vi "TextControlledInstrumCommandsToArraySingle.vi"(10 "SetGetCommands":string, 11 "Control":refnum<vi>) -> (2 "Control to Index":T1(c390), 3 "Command Array":string[][](array[string]))   [LabVIEW 2019]
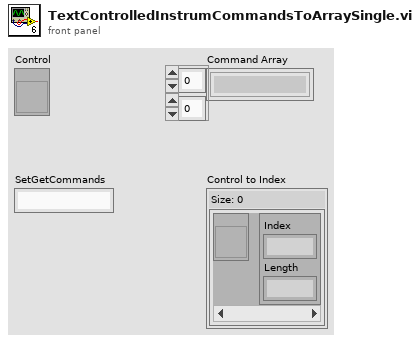
[diagram p1: front panel]
types:
  T1 = map{refnum<vi>, cluster{"Index":i32, "Length":i32}}
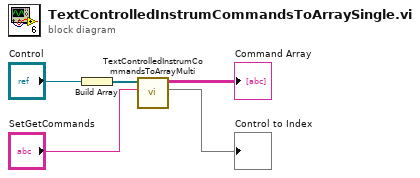
[diagram p0: block diagram]
diagram:
  n1 = Build Array("Control") -> (w4:refnum<vi>[])
  n2 = call "TextControlledInstrumCommandsToArrayMulti.vi"("SetGetCommands"="SetGetCommands", "Control Array"=w4) -> ("Control to Index"=→"Control to Index":T1, "Command Array"=→"Command Array":string[][])  [unwired: 8 in]
